vi "AO Configure Channel.vi"(4 "Blocking (Stream mode)":bool=TRUE, 5 "Samples per channel":dbl=-1.0 format="%#_13g", 6 "Reset index (Periodic mode)":bool=TRUE, 7 "Mode":T1=enum."Stream", 8 "error in (no error)":errorcluster, 9 "Device buffer size":i32=1000, 10 "Sample rate":dbl=1000.0 min=1.0 format="%#_13g", 11 "Analog Output in":refnum<class "Analog output.lvclass">) -> (0 "error out":errorcluster, 3 "Analog Output out":refnum<class "Analog output.lvclass">)   [LabVIEW 2009, in "MicroDAQ.lvlib" / "Analog output.lvclass"]
doc: "Sets the rate of the Sample Clock, and the number of samples to generate (use -1 for continous generation).\nMode options: \nThe periodic mode uses a single buffer which data is output from. When\nthe end of the buffer is reached, data index is switched to the beginning of the buffer. This mode is suitable for generating periodic signals e.g sine waveform. \nThe stream mode uses two buffers architecture to ensure uninterrupted analog signal generation. This mode of operation is suitable for stream data type e.g. generating audio stream, this mode requires from user to queue data with certain time constraints. If new data isn't queued on time, last value remains on analog output until new data has been queued."
uses:
  <instrlib>/MicroDAQ/Channel/Analog Output/Analog output.lvclass
  <instrlib>/MicroDAQ/Tools/Analog mode.ctl
  <instrlib>/MicroDAQ/Channel/Analog Output/Analog output.lvclass/Analog output.ctl
  <instrlib>/MicroDAQ/Mlink library wraper/mlink.lvlib
  <instrlib>/MicroDAQ/MicroDAQ.lvlib
  <instrlib>/MicroDAQ/Channel/Channel.lvclass
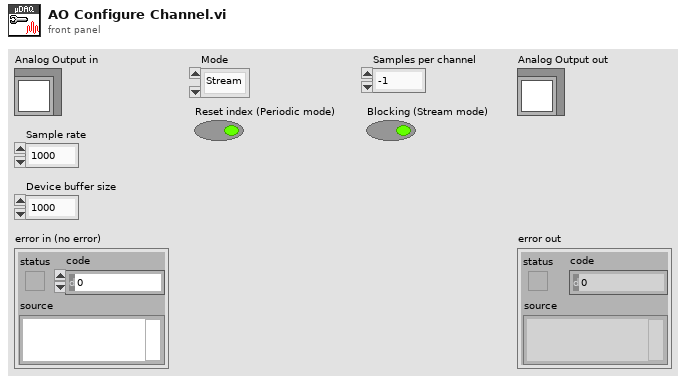
[diagram p1: front panel]
types:
  T1 = typedef "MicroDAQ.lvlib/Analog mode.ctl" = enum16{"Periodic", "Stream"}
  T2 = typedef "MicroDAQ.lvlib/Analo Range Enum.ctl" = enum16{"±10V", "0-10V", "±5V", "0-5V", "±5.12V", "±2.56V", "±2.5V", "±2V", "±1.24V", "±0.64V"}
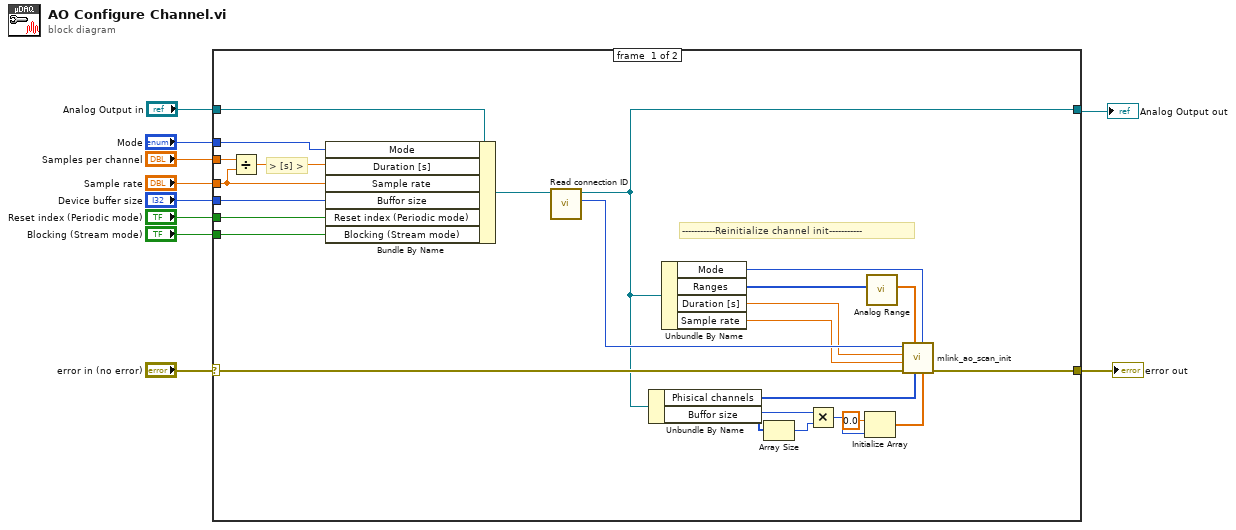
[diagram p0: block diagram]
diagram:
  n1 = case shown="No Error" "error in (no error)" {
    selector: "error in (no error)" -> [w15 w36]
    tunnel: [w16 w36] -> w9
    tunnel: [w11 w35] -> w7
    tunnel: "Analog Output in" -> [w34 w35]
    tunnel: "Mode" -> [w33 _]
    tunnel: "Samples per channel" -> [w29 _]
    tunnel: "Sample rate" -> [w28 _]
    tunnel: "Device buffer size" -> [w32 _]
    tunnel: "Reset index (Periodic mode)" -> [w31 _]
    tunnel: "Blocking (Stream mode)" -> [w30 _]
    frame #0 {
      # "> [s] >"
      # "-----------Reinitialize channel init-----------"
      n2 = Divide(x=w29, y=w28) -> (x/y=w27:dbl)
      n3 = Bundle By Name(cluster=w34, "Mode"=w33, "Duration [s]"=w27, "Sample rate"=w28, "Buffor size"=w32, "Reset index (Periodic mode)"=w31, "Blocking (Stream mode)"=w30) -> (w17:refnum<class "Analog output.lvclass">)
      n4 = call <instrlib>:"Read connection ID.vi"("Task in"=w17) -> ("connection ID"=w14:i32, "Task out"=w11:refnum<class "Analog output.lvclass">)  [unwired: 9 in]
      n5 = Unbundle By Name(w11) -> ("Phisical channels"=w25:u8[], "Buffor size"=w24:i32)
      n6 = Unbundle By Name(w11) -> ("Mode"=w18:T1, "Ranges"=w19:T2[], "Duration [s]"=w13:dbl, "Sample rate"=w12:dbl)
      n7 = Array Size(array=w25) -> (size(s)=w23:i32)
      n8 = Multiply(x=w24, y=w23) -> (x*y=w22:i32)
      n9 = Initialize Array(sgl 0.0 ("element"), w22) -> (w20:sgl[])
      n10 = call <instrlib>:"Analog Range.vi"("ranges in"=w19) -> ("range Array out"=w26:dbl[])  [unwired: 10 in]
      n11 = call <instrlib>:"mlink_ao_scan_init.vi"("data"=w20, "mode"=w18, "channels"=w25, "range"=w26, "error in (no error)"=w15, "rate"=w12, "duration"=w13, "connection ID"=w14) -> ("error out"=w16:errorcluster)  [unwired: 2 in, 1 out]
    }
    frame #1 {
    }
  }
  "error out" <- w9
  "Analog Output out" <- w7
